vi "FindMessages.vi"(7 "BaseActor":refnum<class "BaseActor.lvclass">) -> (3 "Messages":T1)   [LabVIEW 2020, in "jettl.lvlib" / "BaseActor.lvlib" / "BaseActor.lvclass"]
uses:
  BaseActor.lvclass
  BaseActor.lvclass/BaseActor.ctl
  C:/jettl-harness/repos/jettl/src/jettl/jettl/BaseActor/BaseActor/BaseActor.lvclass
  C:/jettl-harness/repos/jettl/src/jettl/jettl/Actor/Actor.lvclass
  jettl.lvlib
  Message/Message.lvclass
  MessageSet.ctl
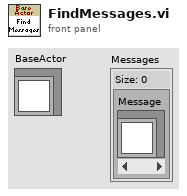
[diagram p1: front panel]
types:
  T1 = typedef "jettl.lvlib/MessageSet.ctl" = set{refnum<class "Message.lvclass">}
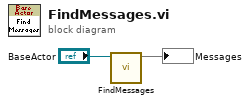
[diagram p0: block diagram]
diagram:
  n1 = call "FindMessages.vi"("{{Name}}Actor.lvclass"="BaseActor") -> ("Messages"=→"Messages":T1)  [unwired: 10 in]
